vi "HDF5_Test3.vi"   [LabVIEW 2018]
uses:
  <vilib>/addons/h5labview2/base/H5Equery.vi
  HDF5/lib_path_mod_20200519.vi
  HDF5/HDF5_ToneInfoClust.ctl
  <vilib>/addons/h5labview2/attrib/H5Awrite.llb/H5Awrite.xnode
  <vilib>/addons/h5labview2/base/hid_t_renamed.ctl
  <vilib>/addons/h5labview2/file/H5F.lvlib
  <vilib>/addons/h5labview2/file/H5Fmode.ctl
  Controls/Clusts/LogLoopClust.ctl
  Controls/ToneInfoClust.ctl
  Controls/Clusts/ChannelToneData.ctl
  Controls/Enums/TargetNumber.ctl
  <vilib>/addons/h5labview2/group/H5G.lvlib
  <vilib>/addons/h5labview2/dataset/H5D.lvlib
  <vilib>/addons/h5labview2/dataset/H5Dwrite.llb/H5Dwrite.xnode
  HDF5/HDF5_Tone_refs.ctl
  HDF5/HDF5_Complex_Refs.ctl
  HDF5/HDF5_ADAM_Refs.ctl
  HDF5/HDF5_Filter_refs.ctl
  HDF5/HDF5_AI_refs.ctl
  Controls/PathsCluster.ctl
  Controls/Enums/ScaleMeasure.ctl
  Controls/Clusts/FPGA_Scale.ctl
  Controls/Clusts/FreqShift.ctl
  Controls/Clusts/FP_UserTargetConfig.ctl
  Controls/Clusts/FrontPanel_UserConfig.ctl
  Controls/Clusts/UserConfig.ctl
  Controls/Clusts/Config_Clust.ctl
  Controls/Clusts/WeatherRefs.ctl
  HDF5/UPS_refs.ctl
  HDF5/HDF5_Health_Refs.ctl
  HDF5/HDF5_Disdrometer_Refs.ctl
  HDF5/HDF5_Validty_refs.ctl
  HDF5/TC_Tone_refs.ctl
  HDF5/HDF5_Noise_refs.ctl
  Controls/Clusts/ToneGroupRefsClust.ctl
  Controls/Clusts/TimeDomainData.ctl
  HDF5/HDF5_ADAM_Data.ctl
  Controls/Clusts/TE_Data_Clust.ctl
  Controls/Clusts/WeatherDataClust.ctl
  Disdrometer/Disdrometer_Status_Cluster.ctl
  HDF5/DisdromterSummaryData.ctl
  HDF5/DisdrometerData.ctl
  HDF5/HDF5_NoiseInfoClust.ctl
  Controls/Clusts/AI_Clust.ctl
  HDF5/TC_Data_Structure.ctl
  Controls/Clusts/ToneLogBuffered.ctl
  Controls/Clusts/LogDataClust.ctl
  Controls/Clusts/HDF5_File_Refs.ctl
  Controls/RadioButtons/FilterEnableRadio.ctl
  Controls/Clusts/Inclinometer_User_Cfg.ctl
  Controls/Clusts/AlarmThresh_OneChan.ctl
  Controls/Clusts/AlarmSettingsClust.ctl
  Controls/Clusts/ErrorStatus.ctl
  Controls/Clusts/ValidityWeatherClust.ctl
  Controls/Clusts/SaturationMonitorBuffer.ctl
  Controls/Clusts/HDF5_10HzRefs.ctl
  Controls/Clusts/Saturation_Status_Clust.ctl
  <vilib>/addons/h5labview2/base/hid_t.ctl
  Controls/Clusts/DigOutClust.ctl
types:
  T1 = typedef "LogLoopClust.ctl" = cluster{"base path":path, "PathNow1":path, "PathNow2":path, "DateNow":string, "NAS path":path, "LogFiltStage":bool, "Config":T2, "HDFRefs1":T13, "HDFRefs2":T13, "LogData":T28, "AlarmCfg":T42, "DO":bool[], "AllAlarms":T44[], "Alarm Status":T45, "SaturationStatus":T46, "WeatherStatus":bool[], "10HzRefs":T47}
  T2 = typedef "Config_Clust.ctl" = cluster{"UsrCfg":T3, "FP_User":T5}
  T3 = typedef "UserConfig.ctl" = cluster{"Paths":T4, "SampleRate":dbl}
  T4 = typedef "PathsCluster.ctl" = cluster{"CfgFile":path, "LogFolder":path, "LogFile":path, "NAS path":path, "ThreshFile":path, "RedunFolder":path}
  T5 = typedef "FrontPanel_UserConfig.ctl" = cluster{"#NoiseSums":u32, "Max_df":u32, "AvgAvg":bool, "#Avg":u16, "AutoCenter":bool, "Inclin":T6, "1":T7, "2":T7, "3":T7, "4":T7, "Target to Probe":T12, "SNR_Thresh":dbl, "Paths":T4, "Connex_Location":string, "SimulateFPGA":bool}
  T6 = typedef "Inclinometer_User_Cfg.ctl" = cluster{"Vmin":dbl, "Vmax":dbl, "Angle_min":dbl, "Angle_max":dbl, "Offset":dbl, "Pos_Neg":bool}
  T7 = typedef "FP_UserTargetConfig.ctl" = cluster{"Cal_":T8, "Beac":T8, "Scale":T9, "Offset":fxp<+/-,16,16>, "Scale_Noise":fxp<+/-,30,30>, "Scale_Step1":fxp<+/-,17,17>, "Scale_In_RT":ext, "ScaleMeas":fxp<+/-,16,1>, "FreqsToRemove":i32[], "Width":i32[], "ScaleMeasEnum":T10, "FilterEnab":T11}
  T8 = typedef "FreqShift.ctl" = cluster{"Fine":dbl, "Coarse_":dbl}
  T9 = typedef "FPGA_Scale.ctl" = cluster{"Step4":fxp<+/-,23,23>, "Step5":fxp<+/-,23,23>, "Step6":fxp<+/-,23,23>, "Step7":fxp<+/-,23,23>}
  T10 = typedef "ScaleMeasure.ctl" = enum16{"1", "10", "50", "42"}
  T11 = typedef "FilterEnableRadio.ctl" = enum32{"None", "Step 1", "Frequency Shift", "Step 4", "Step 5", "Step 6", "Step 7"}
  T12 = typedef "TargetNumber.ctl" = enum16{"1", "2", "3", "4"}
  T13 = typedef "HDF5_File_Refs.ctl" = cluster{"File":T14, "ToneRefs":T15[], "NoiseRefs":T17[], "TC_Refs":T18, "ValidRefs":T19, "DisdromRefs":T20, "TE_Refs":T21, "UPS_Refs_Deprecated":T22, "Weath_Refs":T23, "AI_Refs":T24, "Filter_Refs":T25, "ADAM_Refs":T26, "Complex":T27[]}
  T14 = typedef "hid_t.ctl" = i32
  T15 = typedef "ToneGroupRefsClust.ctl" = cluster{"Group_ref":T14, "Cal":T16, "Beac":T16, "CalZoom_dSet":T14, "BeacZoom_dSet":T14}
  T16 = typedef "HDF5_Tone_refs.ctl" = cluster{"TimeString_dset":T14, "TImeStamp_dset":T14, "SNR_dset":T14, "MaxValue_dset":T14, "PeakLoc_dset":T14, "df_dset":T14, "Phase_dset":T14, "DeltaPhase_dset":T14, "Downshift_dset":T14}
  T17 = typedef "HDF5_Noise_refs.ctl" = cluster{"Group_ref":T14, "TimeString_dset":T14, "TimeStamp_dset":T14, "df_dset":T14, "sum_dset":T14, "SumdSpectrum_dset":T14}
  T18 = typedef "TC_Tone_refs.ctl" = cluster{"Group_ref":T14, "TimeString_dset":T14, "TimeStamp_dset":T14, "TC0_LP1_Hi":T14, "TC1_LP1_MidHi":T14, "TC2_LP1_Mid":T14, "TC3_LP1_LoMid":T14, "TC4_LP1_Lo":T14, "TC5_LP2_Hi":T14, "TC6_LP2_MidHi":T14, "TC7_LP2_Mid":T14, "TC8_LP2_LoMid":T14, "TC9_LP2_Lo":T14, "TC10_HVAC_Cond_In":T14, "TC11_HVAC_Cond_Out":T14, "TC12_Gen_Exhaust":T14, "TC13_Tamb_Inter":T14}
  T19 = typedef "HDF5_Validty_refs.ctl" = cluster{"Group_ref":T14, "Weath_Valid_dset":T14, "Disdr_Valid_dset":T14, "Saturat_dset":T14, "Alarm_Valid_dset":T14, "Time_Valid_dset":T14, "Time_AlarmChange_dset":T14, "Alarm_Source_dset":T14}
  T20 = typedef "HDF5_Disdrometer_Refs.ctl" = cluster{"BasicGroup_ref":T14, "TimeStamp_dset":T14, "TotalRainRate_dset":T14, "Liquid_dset":T14, "Solid_dset":T14, "TotalRain_dset":T14, "Visibility_dset":T14, "RadarReflect_dset":T14, "MaxDiam_dset":T14, "MeasdParticles_dset":T14, "ParticlMinSpeed_dset":T14, "ParticlMaxSpeed_dset":T14, "ParticlMinDiam_dset":T14, "NonHydrParticls_dset":T14, "NonHydrVolum_dset":T14, "UnknownParticls_dset":T14, "UnknownVolum_dset":T14, "HydromType_dset":T14, "SpectGroup_ref":T14, "Spectrum_dset":T14, "Status_dset_deprecated":T14}
  T21 = typedef "HDF5_Health_Refs.ctl" = cluster{"Group_ref":T14, "TE_Temp1_dset":T14, "TE_Outp1_dset":T14, "TE_Temp2_dset":T14, "TE_Outp2_dset":T14, "TE_Temp3_dset":T14, "TE_Outp3_dset":T14, "TimeStamp":T14}
  T22 = typedef "UPS_refs.ctl" = cluster{"Group_ref":T14, "TimeString_dset":T14, "TimeStamp_dset":T14, "V_dset":T14, "A_dset":T14, "Hz_dset":T14, "W_dset":T14, "%_dset":T14}
  T23 = typedef "WeatherRefs.ctl" = cluster{"Group_ref":T14, "TimeString_dset":T14, "TimeStamp_dset ":T14, "WindSpd_dset":T14, "WindGusts_dset":T14, "WindDir_dset":T14, "WindDirSTD_dset":T14, "Temp_dset":T14, "Humidity_dset":T14, "Pressure_dset":T14, "RainRate_dset":T14, "RainFall_dset":T14}
  T24 = typedef "HDF5_AI_refs.ctl" = cluster{"Group_ref":T14, "TimeString_dset":T14, "TimeStamp_dset":T14, "AI0_dset":T14, "AI1_dset":T14, "AI2_dset":T14, "AI3_dset":T14, "AI4_dset":T14, "AI5_dset":T14, "AI6_dset":T14, "AI16_dset":T14, "AI17_dset":T14, "AI18_dset":T14, "AzStdDev_dset":T14, "AI19_dset":T14, "ElStdDev_dset":T14, "BlowerPwr_dset":T14}
  T25 = typedef "HDF5_Filter_refs.ctl" = cluster{"Filter_Group_ref":T14, "TimeStamp_dset":T14, "Filter_dset":T14}
  T26 = typedef "HDF5_ADAM_Refs.ctl" = cluster{"Group_ref":T14, "ADAM_CoPol_dset":T14, "ADAM_XPol_dset":T14, "ADAM_Noise_dset":T14, "ADAM_CalBox_dset":T14, "TimeStamp":T14}
  T27 = typedef "HDF5_Complex_Refs.ctl" = cluster{"Group_ref":T14, "TImeStamp_dset":T14, "PwrSpect_dset":T14, "ISpect_dset":T14, "QSpect_dset":T14}
  T28 = typedef "LogDataClust.ctl" = cluster{"Tone":T29[], "TCData":T31, "AI":T32, "NoiseTrace":cluster{"Target":T12, "NoiseTrace":dbl[]}[], "NoiseInfo":cluster{"Target":T12, "HDF5_NoiseInfo":T33}[], "Disdrom":T34[], "Weath":T37[], "TE":T39, "ADAM":T40, "TimeDomain":T41[]}
  T29 = typedef "ToneLogBuffered.ctl" = cluster{"Count":i32, "CalVal":sgl[], "CalLoc":sgl[], "BeacVal":sgl[], "BeacLoc":sgl[], "BeacShift":sgl[], "Enum":T12, "df":dbl, "PwrSpectr":sgl[][], "ISpectr":sgl[][], "QSpectr":sgl[][], "Time":timestamp[], "SNR":sgl[], "AboveThresh":bool[], "10Hz_PeakVal":dbl[], "Phase":sgl[], "DeltaPhase":dbl[], "Saturat":T30}
  T30 = typedef "SaturationMonitorBuffer.ctl" = cluster{"Meas":bool[], "Stage1":bool[], "Stage4":bool[], "Stage5":bool[], "Stage6":bool[], "Stage7":bool[]}
  T31 = typedef "TC_Data_Structure.ctl" = cluster{"TimeStamp":dbl, "TimeString":string, "TC0_LP1_Hi":dbl, "TC1_LP1_MidHi":dbl, "TC2_LP1_Mid":dbl, "TC3_LP1_LoMid":dbl, "TC4_LP1_Lo":dbl, "TC5_LP2_Hi":dbl, "TC6_LP2_MidHi":dbl, "TC7_LP2_Mid":dbl, "TC8_LP2_LoMid":dbl, "TC9_LP2_Lo":dbl, "TC10_HVAC_Cond_In":dbl, "TC11_HVAC_Cond_Out":dbl, "TC12_Gen_Exhaust":dbl, "TC13_Unused":dbl, "TC14_Unused":dbl, "TC15_Unused":dbl, "TC16_Unused":dbl, "TC17_Unused":dbl, "TC18_Unused":dbl, "TC19_Unused":dbl, "TC20_Unused":dbl, "TC21_Unused":dbl, "TC22_Unused":dbl, "TC23_Unused":dbl, "TC24_Unused":dbl, "TC25_Unused":dbl, "TC26_Unused":dbl, "TC27_Unused":dbl, "TC28_Unused":dbl, "TC29_Unused":dbl, "TC30_Unused":dbl, "TC31_Unused":dbl}
  T32 = typedef "AI_Clust.ctl" = cluster{"TimeString":string, "Time Stamp":dbl, "AI0_Unused":dbl, "AI1_-5V":dbl, "AI2_+5V":dbl, "AI3_+6V":dbl, "AI4_+12V":dbl, "AI5_+15V":dbl, "AI6_+28V":dbl, "AI7_Unused":dbl, "Ai16_72GHz_CalPower":dbl, "Ai17_84GHz_CalPower":dbl, "Ai18_InclinAz":dbl, "Ai19_InclinEl":dbl, "Ai20_BlowerPwr":dbl, "Ai21_Unused":dbl, "Ai22_Unused":dbl, "Ai23_Unused":dbl, "InclinA_StdDev":dbl, "InclinB_StdDev":dbl, "InclinAz_Unfilt":dbl, "InclinEl_Unfilt":dbl}
  T33 = typedef "HDF5_NoiseInfoClust.ctl" = cluster{"Timestring":string, "Timestamp":dbl, "df":dbl, "Sum":dbl}
  T34 = typedef "DisdrometerData.ctl" = cluster{"Spectrum Data":i16[], "DisdromSummary":T35, "Status":T36}
  T35 = typedef "DisdromterSummaryData.ctl" = cluster{"current time":dbl, "Timestamp":dbl, "Total Rain Rate":dbl, "Liquid Rain Rate":dbl, "Solid Rain Rate":dbl, "Total Rainfall":dbl, "Visibility":dbl, "Radar Reflectivity":dbl, "Max Diameter Hail":dbl, "Measured Particles":i16, "Particle Min Speed":i16, "Particle Max Speed":i16, "Particle Min Diam":i16, "NonHydr Particles":i16, "NonHydr Volume":dbl, "Unkn Particles":i16, "Unkn Volume":dbl, "HydroType":i8}
  T36 = typedef "Disdrometer_Status_Cluster.ctl" = cluster{"Laser":bool, "Signal":bool, "LaserTemp_Analog":bool, "LaserTemp_Digital":bool, "LaserCurrent_Analog":bool, "LaserCurrent_Digital":bool, "SensorSupply":bool, "HeatLaserHead":bool, "HeatReceiverHead":bool, "TempSensor":bool, "HeatSupply":bool, "HeatHousing":bool, "HeatHeads":bool, "HeatCarriers":bool, "OutputLaserPower":bool, "Checksum":bool, "StatusInt":u16}
  T37 = typedef "WeatherDataClust.ctl" = cluster{"TimeString":string, "Timestamp":dbl, "Wind Speed":sgl, "Wind Gusts":sgl, "Wind Dir":sgl, "Wind Dir STD":sgl, "Temperature":sgl, "Humidity":sgl, "Pressure":sgl, "Rain Rate":i16, "Rain Fall":sgl, "Status":T38}
  T38 = typedef "ValidityWeatherClust.ctl" = cluster{"Temp_OutOfBounds":bool, "Temp_IncrSTD":bool, "Temp_Oth":bool, "BarPress_OutOfBounds":bool, "BarPress_IncrSTD":bool, "BarPress_Change":bool, "BarPress_Other":bool, "Humid_OutOfBounds":bool, "Humid_IncrSTD":bool, "Humid_Other":bool, "Wind__Spd_OutOfBounds":bool, "Wind_Dir_OutOfBounds":bool, "RainBuck_OutOfBounds":bool, "RainBuck_Disdrom":bool, "Disdrom_RainBuck":bool, "Placeholder":bool}
  T39 = typedef "TE_Data_Clust.ctl" = cluster{"TimeString":string, "TimeStamp":dbl, "Temp":dbl, "Output":dbl, "Temp 2":dbl, "Output 2":dbl, "Temp 3":dbl, "Output 3":dbl}
  T40 = typedef "HDF5_ADAM_Data.ctl" = cluster{"Timestamp":dbl, "Time string":string, "Fault 1":bool, "Fault 2":bool, "Fault 3":bool, "Fault 4":bool, "Fault 5":bool, "Fault 6":bool, "Value 1":dbl, "Value 2":dbl, "Value 3":dbl, "Value 4":dbl, "Value 5":dbl, "Value 6":dbl}
  T41 = typedef "TimeDomainData.ctl" = cluster{"CalTimeVal":dbl[], "CalTimeCount":u32[], "Enum":T12}
  T42 = typedef "AlarmSettingsClust.ctl" = cluster{"TC13":T43, "AI1":T43, "AI2":T43, "AI3":T43, "AI4":T43, "AI5":T43, "AI6":T43, "AI18":T43, "AI19":T43, "TE1":T43, "TE2":T43, "TE3":T43, "ADAM1":T43, "ADAM2":T43, "ADAM3":T43, "ADAM4":T43, "72CoBeacFreq":T43, "72CoCalFreq":T43, "84CoBeacFreq":T43, "84CoCalFreq":T43, "72Co_CalTonePwr":T43, "72X_CalTonePwr":T43, "84Co_CalTonePwr":T43, "84X_CalTonePwr":T43}
  T43 = typedef "AlarmThresh_OneChan.ctl" = cluster{"Enbl":bool, "ErrsAndWarns":cluster{dbl, dbl, dbl, dbl}}
  T44 = typedef "ErrorStatus.ctl" = cluster{"RX?":bool, "Warn":bool, "Error":bool, "Enabl":bool, "Source":string}
  T45 = typedef "DigOutClust.ctl" = cluster{"Green":bool, "Rx_Yell":bool, "Cx_Yell":bool, "Red":bool, "Source":string}
  T46 = typedef "Saturation_Status_Clust.ctl" = cluster{"84":bool[], "72":bool[]}
  T47 = typedef "HDF5_10HzRefs.ctl" = cluster{"72Co_dset":T14, "84Co_dset":T14, "FileRef":T14}
  T48 = typedef "H5F.lvlib/H5Fmode.ctl" = enum16{"read-only", "read-write", "overwrite", "create new", "open or create"}
  T49 = typedef "ChannelToneData.ctl" = cluster{"LastPk":dbl, "Shift_":dbl, "Pk_PreShift":dbl, "Peak_ToFPGA":dbl, "MaxValue":dbl, "MaxIndex":i32, "Tone":T50, "TimeDomainI":ext[], "TimeDomainQ":ext[], "PwrSpectrum":dbl[], "RunningAvgFreq":dbl, "PhaseSpect":dbl[], "RealSpect":dbl[], "ImagSpect":dbl[]}
  T50 = typedef "ToneInfoClust.ctl" = cluster{"PeakLoc":dbl, "df_":dbl, "ZoomPwr":dbl[], "ZoomPhase":dbl[]}
  T51 = typedef "HDF5_ToneInfoClust.ctl" = cluster{"Timestring":string, "Timestamp":dbl, "MaxValue":dbl, "PeakLoc":dbl, "df":dbl}
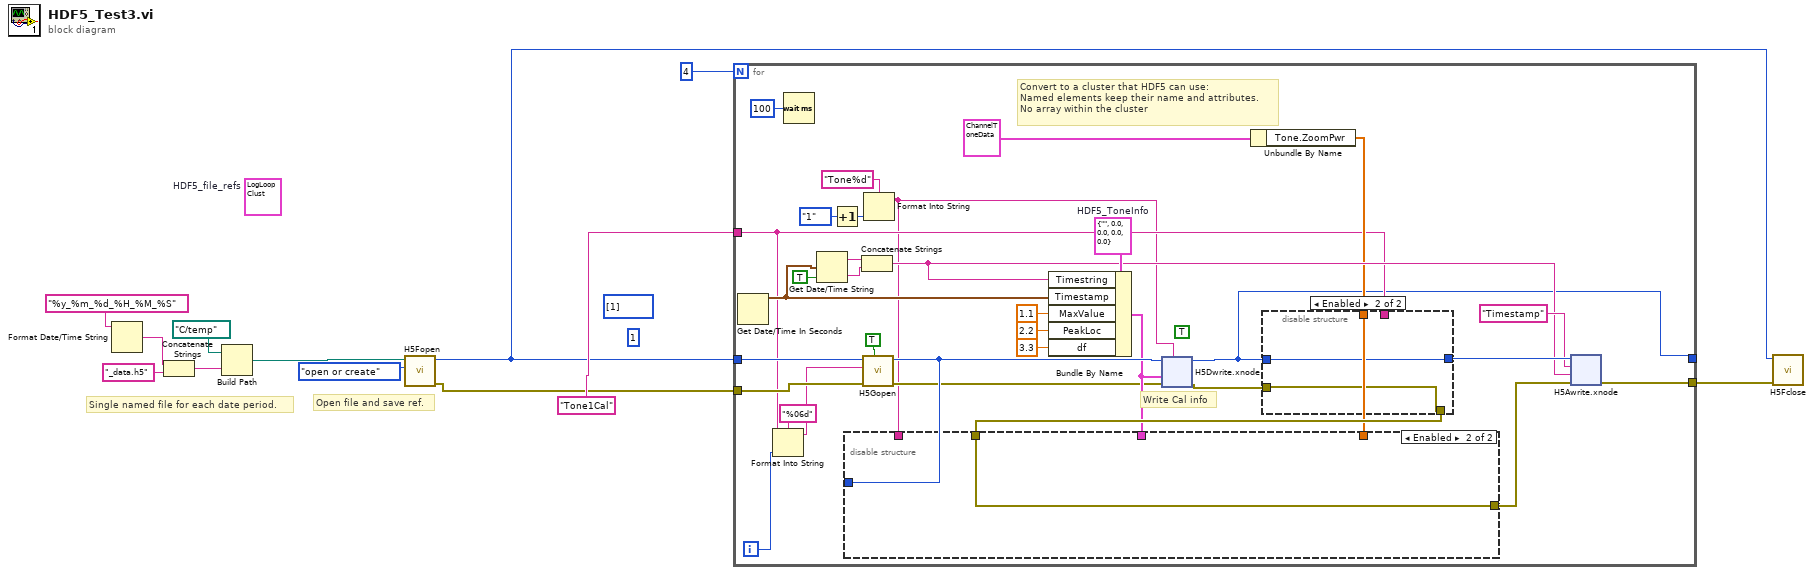
[diagram p0: block diagram]
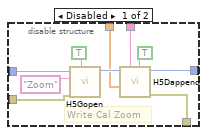
[diagram p2: hidden frame]
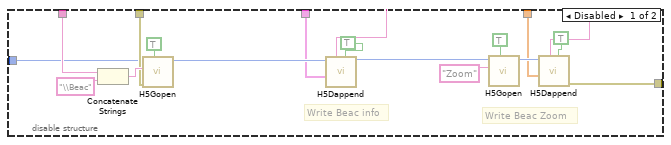
[diagram p3: hidden frame]
diagram:
  (unwired) 1 ("ndims")
  (unwired) u64[] [1] ("chunk size")
  (unwired) T1 {"base path"=path "", "PathNow1"=path "", "PathNow2"=path "", "DateNow"="", "NAS path"=path "", "LogFiltStage"=FALSE, "Config"={"UsrCfg"={"Paths"={"CfgFile"=path "", "LogFolder"=path "", "LogFile"=path "", "NAS path"=path "", "ThreshFile"=path "", "RedunFolder"=path ""}, "SampleRate"=0.0}, "FP_User"={"#NoiseSums"=0, "Max_df"=0, "AvgAvg"=FALSE, "#Avg"=0, "AutoCenter"=FALSE, "Inclin"={"Vmin"=0.0, "Vmax"=0.0, "Angle_min"=0.0, "Angle_max"=0.0, "Offset"=0.0, "Pos_Neg"=FALSE}, "1"={"Cal_"={"Fine"=0.0, "Coarse_"=0.0}, "Beac"={"Fine"=0.0, "Coarse_"=0.0}, "Scale"={"Step4"=0.0, "Step5"=0.0, "Step6"=0.0, "Step7"=0.0}, "Offset"=0.0, "Scale_Noise"=0.0, "Scale_Step1"=0.0, "Scale_In_RT"=0.0, "ScaleMeas"=0.0, "FreqsToRemove"=[], "Width"=[], "ScaleMeasEnum"=enum."1", "FilterEnab"=enum."None"}, "2"={"Cal_"={"Fine"=0.0, "Coarse_"=0.0}, "Beac"={"Fine"=0.0, "Coarse_"=0.0}, "Scale"={"Step4"=0.0, "Step5"=0.0, "Step6"=0.0, "Step7"=0.0}, "Offset"=0.0, "Scale_Noise"=0.0, "Scale_Step1"=0.0, "Scale_In_RT"=0.0, "ScaleMeas"=0.0, "FreqsToRemove"=[], "Width"=[], "ScaleMeasEnum"=enum."1", "FilterEnab"=enum."None"}, "3"={"Cal_"={"Fine"=0.0, "Coarse_"=0.0}, "Beac"={"Fine"=0.0, "Coarse_"=0.0}, "Scale"={"Step4"=0.0, "Step5"=0.0, "Step6"=0.0, "Step7"=0.0}, "Offset"=0.0, "Scale_Noise"=0.0, "Scale_Step1"=0.0, "Scale_In_RT"=0.0, "ScaleMeas"=0.0, "FreqsToRemove"=[], "Width"=[], "ScaleMeasEnum"=enum."1", "FilterEnab"=enum."None"}, "4"={"Cal_"={"Fine"=0.0, "Coarse_"=0.0}, "Beac"={"Fine"=0.0, "Coarse_"=0.0}, "Scale"={"Step4"=0.0, "Step5"=0.0, "Step6"=0.0, "Step7"=0.0}, "Offset"=0.0, "Scale_Noise"=0.0, "Scale_Step1"=0.0, "Scale_In_RT"=0.0, "ScaleMeas"=0.0, "FreqsToRemove"=[], "Width"=[], "ScaleMeasEnum"=enum."1", "FilterEnab"=enum."None"}, "Target to Probe"=enum."1", "SNR_Thresh"=0.0, "Paths"={"CfgFile"=path "", "LogFolder"=path "", "LogFile"=path "", "NAS path"=path "", "ThreshFile"=path "", "RedunFolder"=path ""}, "Connex_Location"="", "SimulateFPGA"=FALSE}}, "HDFRefs1"={"File"=0, "ToneRefs"=[], "NoiseRefs"=[], "TC_Refs"={"Group_ref"=0, "TimeString_dset"=0, "TimeStamp_dset"=0, "TC0_LP1_Hi"=0, "TC1_LP1_MidHi"=0, "TC2_LP1_Mid"=0, "TC3_LP1_LoMid"=0, "TC4_LP1_Lo"=0, "TC5_LP2_Hi"=0, "TC6_LP2_MidHi"=0, "TC7_LP2_Mid"=0, "TC8_LP2_LoMid"=0, "TC9_LP2_Lo"=0, "TC10_HVAC_Cond_In"=0, "TC11_HVAC_Cond_Out"=0, "TC12_Gen_Exhaust"=0, "TC13_Tamb_Inter"=0}, "ValidRefs"={"Group_ref"=0, "Weath_Valid_dset"=0, "Disdr_Valid_dset"=0, "Saturat_dset"=0, "Alarm_Valid_dset"=0, "Time_Valid_dset"=0, "Time_AlarmChange_dset"=0, "Alarm_Source_dset"=0}, "DisdromRefs"={"BasicGroup_ref"=0, "TimeStamp_dset"=0, "TotalRainRate_dset"=0, "Liquid_dset"=0, "Solid_dset"=0, "TotalRain_dset"=0, "Visibility_dset"=0, "RadarReflect_dset"=0, "MaxDiam_dset"=0, "MeasdParticles_dset"=0, "ParticlMinSpeed_dset"=0, "ParticlMaxSpeed_dset"=0, "ParticlMinDiam_dset"=0, "NonHydrParticls_dset"=0, "NonHydrVolum_dset"=0, "UnknownParticls_dset"=0, "UnknownVolum_dset"=0, "HydromType_dset"=0, "SpectGroup_ref"=0, "Spectrum_dset"=0, "Status_dset_deprecated"=0}, "TE_Refs"={"Group_ref"=0, "TE_Temp1_dset"=0, "TE_Outp1_dset"=0, "TE_Temp2_dset"=0, "TE_Outp2_dset"=0, "TE_Temp3_dset"=0, "TE_Outp3_dset"=0, "TimeStamp"=0}, "UPS_Refs_Deprecated"={"Group_ref"=0, "TimeString_dset"=0, "TimeStamp_dset"=0, "V_dset"=0, "A_dset"=0, "Hz_dset"=0, "W_dset"=0, "%_dset"=0}, "Weath_Refs"={"Group_ref"=0, "TimeString_dset"=0, "TimeStamp_dset "=0, "WindSpd_dset"=0, "WindGusts_dset"=0, "WindDir_dset"=0, "WindDirSTD_dset"=0, "Temp_dset"=0, "Humidity_dset"=0, "Pressure_dset"=0, "RainRate_dset"=0, "RainFall_dset"=0}, "AI_Refs"={"Group_ref"=0, "TimeString_dset"=0, "TimeStamp_dset"=0, "AI0_dset"=0, "AI1_dset"=0, "AI2_dset"=0, "AI3_dset"=0, "AI4_dset"=0, "AI5_dset"=0, "AI6_dset"=0, "AI16_dset"=0, "AI17_dset"=0, "AI18_dset"=0, "AzStdDev_dset"=0, "AI19_dset"=0, "ElStdDev_dset"=0, "BlowerPwr_dset"=0}, "Filter_Refs"={"Filter_Group_ref"=0, "TimeStamp_dset"=0, "Filter_dset"=0}, "ADAM_Refs"={"Group_ref"=0, "ADAM_CoPol_dset"=0, "ADAM_XPol_dset"=0, "ADAM_Noise_dset"=0, "ADAM_CalBox_dset"=0, "TimeStamp"=0}, "Complex"=[]}, "HDFRefs2"={"File"=0, "ToneRefs"=[], "NoiseRefs"=[], "TC_Refs"={"Group_ref"=0, "TimeString_dset"=0, "TimeStamp_dset"=0, "TC0_LP1_Hi"=0, "TC1_LP1_MidHi"=0, "TC2_LP1_Mid"=0, "TC3_LP1_LoMid"=0, "TC4_LP1_Lo"=0, "TC5_LP2_Hi"=0, "TC6_LP2_MidHi"=0, "TC7_LP2_Mid"=0, "TC8_LP2_LoMid"=0, "TC9_LP2_Lo"=0, "TC10_HVAC_Cond_In"=0, "TC11_HVAC_Cond_Out"=0, "TC12_Gen_Exhaust"=0, "TC13_Tamb_Inter"=0}, "ValidRefs"={"Group_ref"=0, "Weath_Valid_dset"=0, "Disdr_Valid_dset"=0, "Saturat_dset"=0, "Alarm_Valid_dset"=0, "Time_Valid_dset"=0, "Time_AlarmChange_dset"=0, "Alarm_Source_dset"=0}, "DisdromRefs"={"BasicGroup_ref"=0, "TimeStamp_dset"=0, "TotalRainRate_dset"=0, "Liquid_dset"=0, "Solid_dset"=0, "TotalRain_dset"=0, "Visibility_dset"=0, "RadarReflect_dset"=0, "MaxDiam_dset"=0, "MeasdParticles_dset"=0, "ParticlMinSpeed_dset"=0, "ParticlMaxSpeed_dset"=0, "ParticlMinDiam_dset"=0, "NonHydrParticls_dset"=0, "NonHydrVolum_dset"=0, "UnknownParticls_dset"=0, "UnknownVolum_dset"=0, "HydromType_dset"=0, "SpectGroup_ref"=0, "Spectrum_dset"=0, "Status_dset_deprecated"=0}, "TE_Refs"={"Group_ref"=0, "TE_Temp1_dset"=0, "TE_Outp1_dset"=0, "TE_Temp2_dset"=0, "TE_Outp2_dset"=0, "TE_Temp3_dset"=0, "TE_Outp3_dset"=0, "TimeStamp"=0}, "UPS_Refs_Deprecated"={"Group_ref"=0, "TimeString_dset"=0, "TimeStamp_dset"=0, "V_dset"=0, "A_dset"=0, "Hz_dset"=0, "W_dset"=0, "%_dset"=0}, "Weath_Refs"={"Group_ref"=0, "TimeString_dset"=0, "TimeStamp_dset "=0, "WindSpd_dset"=0, "WindGusts_dset"=0, "WindDir_dset"=0, "WindDirSTD_dset"=0, "Temp_dset"=0, "Humidity_dset"=0, "Pressure_dset"=0, "RainRate_dset"=0, "RainFall_dset"=0}, "AI_Refs"={"Group_ref"=0, "TimeString_dset"=0, "TimeStamp_dset"=0, "AI0_dset"=0, "AI1_dset"=0, "AI2_dset"=0, "AI3_dset"=0, "AI4_dset"=0, "AI5_dset"=0, "AI6_dset"=0, "AI16_dset"=0, "AI17_dset"=0, "AI18_dset"=0, "AzStdDev_dset"=0, "AI19_dset"=0, "ElStdDev_dset"=0, "BlowerPwr_dset"=0}, "Filter_Refs"={"Filter_Group_ref"=0, "TimeStamp_dset"=0, "Filter_dset"=0}, "ADAM_Refs"={"Group_ref"=0, "ADAM_CoPol_dset"=0, "ADAM_XPol_dset"=0, "ADAM_Noise_dset"=0, "ADAM_CalBox_dset"=0, "TimeStamp"=0}, "Complex"=[]}, "LogData"={"Tone"=[], "TCData"={"TimeStamp"=0.0, "TimeString"="", "TC0_LP1_Hi"=0.0, "TC1_LP1_MidHi"=0.0, "TC2_LP1_Mid"=0.0, "TC3_LP1_LoMid"=0.0, "TC4_LP1_Lo"=0.0, "TC5_LP2_Hi"=0.0, "TC6_LP2_MidHi"=0.0, "TC7_LP2_Mid"=0.0, "TC8_LP2_LoMid"=0.0, "TC9_LP2_Lo"=0.0, "TC10_HVAC_Cond_In"=0.0, "TC11_HVAC_Cond_Out"=0.0, "TC12_Gen_Exhaust"=0.0, "TC13_Unused"=0.0, "TC14_Unused"=0.0, "TC15_Unused"=0.0, "TC16_Unused"=0.0, "TC17_Unused"=0.0, "TC18_Unused"=0.0, "TC19_Unused"=0.0, "TC20_Unused"=0.0, "TC21_Unused"=0.0, "TC22_Unused"=0.0, "TC23_Unused"=0.0, "TC24_Unused"=0.0, "TC25_Unused"=0.0, "TC26_Unused"=0.0, "TC27_Unused"=0.0, "TC28_Unused"=0.0, "TC29_Unused"=0.0, "TC30_Unused"=0.0, "TC31_Unused"=0.0}, "AI"={"TimeString"="", "Time Stamp"=0.0, "AI0_Unused"=0.0, "AI1_-5V"=0.0, "AI2_+5V"=0.0, "AI3_+6V"=0.0, "AI4_+12V"=0.0, "AI5_+15V"=0.0, "AI6_+28V"=0.0, "AI7_Unused"=0.0, "Ai16_72GHz_CalPower"=0.0, "Ai17_84GHz_CalPower"=0.0, "Ai18_InclinAz"=0.0, "Ai19_InclinEl"=0.0, "Ai20_BlowerPwr"=0.0, "Ai21_Unused"=0.0, "Ai22_Unused"=0.0, "Ai23_Unused"=0.0, "InclinA_StdDev"=0.0, "InclinB_StdDev"=0.0, "InclinAz_Unfilt"=0.0, "InclinEl_Unfilt"=0.0}, "NoiseTrace"=[], "NoiseInfo"=[], "Disdrom"=[], "Weath"=[], "TE"={"TimeString"="", "TimeStamp"=0.0, "Temp"=0.0, "Output"=0.0, "Temp 2"=0.0, "Output 2"=0.0, "Temp 3"=0.0, "Output 3"=0.0}, "ADAM"={"Timestamp"=0.0, "Time string"="", "Fault 1"=FALSE, "Fault 2"=FALSE, "Fault 3"=FALSE, "Fault 4"=FALSE, "Fault 5"=FALSE, "Fault 6"=FALSE, "Value 1"=0.0, "Value 2"=0.0, "Value 3"=0.0, "Value 4"=0.0, "Value 5"=0.0, "Value 6"=0.0}, "TimeDomain"=[]}, "AlarmCfg"={"TC13"={"Enbl"=FALSE, "ErrsAndWarns"={0.0, 0.0, 0.0, 0.0}}, "AI1"={"Enbl"=FALSE, "ErrsAndWarns"={0.0, 0.0, 0.0, 0.0}}, "AI2"={"Enbl"=FALSE, "ErrsAndWarns"={0.0, 0.0, 0.0, 0.0}}, "AI3"={"Enbl"=FALSE, "ErrsAndWarns"={0.0, 0.0, 0.0, 0.0}}, "AI4"={"Enbl"=FALSE, "ErrsAndWarns"={0.0, 0.0, 0.0, 0.0}}, "AI5"={"Enbl"=FALSE, "ErrsAndWarns"={0.0, 0.0, 0.0, 0.0}}, "AI6"={"Enbl"=FALSE, "ErrsAndWarns"={0.0, 0.0, 0.0, 0.0}}, "AI18"={"Enbl"=FALSE, "ErrsAndWarns"={0.0, 0.0, 0.0, 0.0}}, "AI19"={"Enbl"=FALSE, "ErrsAndWarns"={0.0, 0.0, 0.0, 0.0}}, "TE1"={"Enbl"=FALSE, "ErrsAndWarns"={0.0, 0.0, 0.0, 0.0}}, "TE2"={"Enbl"=FALSE, "ErrsAndWarns"={0.0, 0.0, 0.0, 0.0}}, "TE3"={"Enbl"=FALSE, "ErrsAndWarns"={0.0, 0.0, 0.0, 0.0}}, "ADAM1"={"Enbl"=FALSE, "ErrsAndWarns"={0.0, 0.0, 0.0, 0.0}}, "ADAM2"={"Enbl"=FALSE, "ErrsAndWarns"={0.0, 0.0, 0.0, 0.0}}, "ADAM3"={"Enbl"=FALSE, "ErrsAndWarns"={0.0, 0.0, 0.0, 0.0}}, "ADAM4"={"Enbl"=FALSE, "ErrsAndWarns"={0.0, 0.0, 0.0, 0.0}}, "72CoBeacFreq"={"Enbl"=FALSE, "ErrsAndWarns"={0.0, 0.0, 0.0, 0.0}}, "72CoCalFreq"={"Enbl"=FALSE, "ErrsAndWarns"={0.0, 0.0, 0.0, 0.0}}, "84CoBeacFreq"={"Enbl"=FALSE, "ErrsAndWarns"={0.0, 0.0, 0.0, 0.0}}, "84CoCalFreq"={"Enbl"=FALSE, "ErrsAndWarns"={0.0, 0.0, 0.0, 0.0}}, "72Co_CalTonePwr"={"Enbl"=FALSE, "ErrsAndWarns"={0.0, 0.0, 0.0, 0.0}}, "72X_CalTonePwr"={"Enbl"=FALSE, "ErrsAndWarns"={0.0, 0.0, 0.0, 0.0}}, "84Co_CalTonePwr"={"Enbl"=FALSE, "ErrsAndWarns"={0.0, 0.0, 0.0, 0.0}}, "84X_CalTonePwr"={"Enbl"=FALSE, "ErrsAndWarns"={0.0, 0.0, 0.0, 0.0}}}, "DO"=[], "AllAlarms"=[], "Alarm Status"={"Green"=FALSE, "Rx_Yell"=FALSE, "Cx_Yell"=FALSE, "Red"=FALSE, "Source"=""}, "SaturationStatus"={"84"=[], "72"=[]}, "WeatherStatus"=[], "10HzRefs"={"72Co_dset"=0, "84Co_dset"=0, "FileRef"=0}}  # HDF5_file_refs
  # "Open file and save ref."
  # "Single named file for each date period."
  n1 = Format Date/Time String(time format string (%c)="%y_%m_%d_%H_%M_%S") -> (date/time string=w7:string)  [unwired: 2 in]
  n2 = Concatenate Strings(w7, "_data.h5" ("string")) -> (w11:string)
  n3 = Build Path(base path=path "C:/temp", name or relative path=w11) -> (appended path=w9:path)
  n4 = call <vilib>:"H5Fopen.vi"("mode (read-only)"=H5Fmode."open or create", "path"=w9) -> ("error out"=w2:errorcluster, "ref out"=w3:T14)  [unwired: 8 in]
  n5 = for {
    N: 4 -> [_]
    tunnel: w3 -> [w25]
    tunnel: [w18] -> _
    tunnel: [w26] -> w1
    tunnel: "Tone1Cal" ("name") -> [w22]
    tunnel: w2 -> [w24]
    i -> [w23]
    (unwired) TRUE ("create? (T)")
    w44 = T51 {"Timestring"="", "Timestamp"=0.0, "MaxValue"=0.0, "PeakLoc"=0.0, "df"=0.0}  # HDF5_ToneInfo
    # "Write Cal info"
    # "Convert to a cluster that HDF5 can use:\nNamed elements keep their name and attributes.\nNo array within the cluster"
    n6 = Get Date/Time In Seconds() -> (seconds since 1Jan1904=w32:timestamp)
    n7 = Format Into String(format string="%06d", initial string=w22, w23) -> (resulting string=w20:string)  [unwired: 1 in, 1 out]
    n8 = Wait (ms)(milliseconds to wait=u32 100) -> ()  [unwired: 1 out]
    n9 = Get Date/Time String(seconds (now)=w32, want seconds? (F)=TRUE) -> (date string=w35:string, time string=w34:string)  [unwired: 1 in]
    n10 = Increment(x=TargetNumber."1" ("input 1")) -> (x+1=w27:T12)
    n11 = Concatenate Strings(w35, w34) -> (w33:string)
    n12 = call <vilib>:"H5Gopen.vi"("create? (F)"=TRUE, "error in (no error)"=w24, "name"=w20, "ref in"=w25) -> ("error out"=w14:errorcluster, "group out"=w19:T14)  [unwired: 6 in]
    n13 = Format Into String(format string="Tone%d", w27) -> (resulting string=w13:string)  [unwired: 2 in, 1 out]
    n14 = Bundle By Name(cluster=w44, "Timestring"=w33, "Timestamp"=w32, "MaxValue"=1.1, "PeakLoc"=2.2 ("MaxValue"), "df"=3.3 ("MaxValue")) -> (w17:T51)
    n15 = xnode "H5Dwrite.xnode"("dataset name"=w13, "error in (no error)"=w14, "data"=w17, "ref in"=w19) -> ("error out"=w16:errorcluster, "ref out"=w18:i32)  [unwired: 3 in, 1 out]
    n16 = Unbundle By Name(T49 {"LastPk"=0.0, "Shift_"=-24999462.633451957, "Pk_PreShift"=0.0, "Peak_ToFPGA"=-24999462.633451957, "MaxValue"=0.0, "MaxIndex"=0, "Tone"={"PeakLoc"=0.0, "df_"=0.0, "ZoomPwr"=[0.0, 0.0, 0.0, 0.0, 0.0, 0.0, 0.0, 0.0, 8.8, 9.9, 10.1], "ZoomPhase"=[]}, "TimeDomainI"=array[12500 elements], "TimeDomainQ"=[], "PwrSpectrum"=[], "RunningAvgFreq"=0.0, "PhaseSpect"=[], "RealSpect"=[], "ImagSpect"=[]} ("input cluster")) -> ("Tone.ZoomPwr"=w30:dbl[])
    n17 = disable-structure shown="Enabled" {
      disable-tunnel: [w74 w76] -> w43
      disable-tunnel: [w70 w75] -> w31
      disable-tunnel: w30 -> [w69 _]
      disable-tunnel: w18 -> [w67 w76]
      disable-tunnel: w22 -> [w66 _]
      disable-tunnel: w16 -> [w65 w75]
      frame Disabled {
        # "Write Cal Zoom"
        n18 = call <vilib>:"H5Gopen.vi"("create? (F)"=TRUE, "error in (no error)"=w65, "name"="Zoom", "ref in"=w67) -> ("group out"=w71:T14)  [unwired: 6 in, 1 out]
        n19 = call <vilib>:"H5Dappend.vi"("create? (T)"=TRUE, "dataset name"=w66, "data"=w69, "ref in"=w71) -> ("error out"=w70:errorcluster, "ref out"=w74:T14)  [unwired: 4 in, 2 out]
      }
      frame Enabled {
      }
    }
    n20 = disable-structure shown="Enabled" {
      disable-tunnel: w31 -> [w87 w93]
      disable-tunnel: w17 -> [w86 _]
      disable-tunnel: w30 -> [w82 _]
      disable-tunnel: [w81 w93] -> w29
      disable-tunnel: w13 -> [w80 _]
      disable-tunnel: w19 -> [w77 _]
      frame Disabled {
        # "Write Beac Zoom"
        # "Write Beac info"
        n21 = Concatenate Strings(w80, "\\Beac" ("string")) -> (w90:string)
        n22 = call <vilib>:"H5Gopen.vi"("create? (F)"=TRUE, "error in (no error)"=w87, "name"=w90, "ref in"=w77) -> ("group out"=w88:T14)  [unwired: 6 in, 1 out]
        n23 = call <vilib>:"H5Dappend.vi"("create? (T)"=TRUE, "dataset name"=w80, "data"=w86, "ref in"=w88) -> ("ref out"=w85:T14)  [unwired: 4 in, 3 out]
        n24 = call <vilib>:"H5Gopen.vi"("create? (F)"=TRUE, "name"="Zoom", "ref in"=w85) -> ("group out"=w83:T14)  [unwired: 7 in, 1 out]
        n25 = call <vilib>:"H5Dappend.vi"("create? (T)"=TRUE, "dataset name"=w80, "data"=w82, "ref in"=w83) -> ("error out"=w81:errorcluster)  [unwired: 4 in, 3 out]
      }
      frame Enabled {
      }
    }
    n26 = xnode "H5Awrite.xnode"("error in (no error)"=w29, "data"=w33, "attrib name"="Timestamp" ("delimiter (Tab)"), "ref in"=w43) -> ("error out"=w26:errorcluster)  [unwired: 3 in, 2 out]
  }
  n27 = call <vilib>:"H5Fclose.vi"("error in (no error)"=w1, "ref"=w3) -> ()  [unwired: 9 in, 1 out]
